vi "Main.vi"(11 "Module Admin":refnum<class "Delacor_lib_QMH_Module Admin.lvclass">) -> ()   [LabVIEW 2019, in "UI.lvlib"]
doc: "This template is based off of the Queued Message Handler design pattern and the Queued Message Handler project template that ships with LabVIEW.\n\nThe main difference is that the queue is private to this module and communication between modules is performed via Broadcast and Request events.\n\nRequest events are wrapped in public API methods and are handled in the Event Handling Loop (EHL) of this VI. Any module can register for Broadcast events sent by this module. The EHL generates messages based on user interface actions.\n\nThe Message Handling Loop (MHL) processes messages generated by the EHL, or by other messages. The messages are string values, so new messages can be added easily to the Message Cases case structure in the MHL. Each message cluster can also provide an optional value for Message Data, which is a variant that can be converted to whatever message-specific data is required.\n_____\nBased on Delacor QMH Project Template 5.0.0.82."
uses:
  UI.lvlib
  <vilib>/Delacor/Delacor QMH/Libraries/Module Admin_class/Delacor_lib_QMH_Module Admin.lvclass
  Module Data--cluster.ctl
  Stop Argument--cluster.ctl
  <vilib>/Delacor/Delacor QMH/Libraries/Message Queue_class/Delacor_lib_QMH_Message Queue.lvclass/Delacor_lib_QMH_Message Queue.ctl
  <vilib>/Delacor/Delacor QMH/Libraries/Module Admin_class/Delacor_lib_QMH_Module Admin.lvclass/Delacor_lib_QMH_Module Admin.ctl
  <vilib>/Delacor/Delacor QMH/Libraries/Message Queue_class/Delacor_lib_QMH_Enqueue Message (Single).vi
  <vilib>/Delacor/Delacor QMH/Libraries/Module Admin_class/Delacor_lib_QMH_Get External Launch.vi
  <vilib>/Utility/error.llb/Error Cluster From Error Code.vi
  <vilib>/ErrorRing/Error Ring.xnode
  <vilib>/Delacor/Delacor QMH/Libraries/Message Queue_class/Delacor_lib_QMH_Message Queue.lvclass
  Adquisition/Adquisition.lvlib
  Analisis/Analisis.lvlib
  Mensajes/Mensajes .lvlib
  config/config.lvlib
panel:
  out "error out":errorcluster
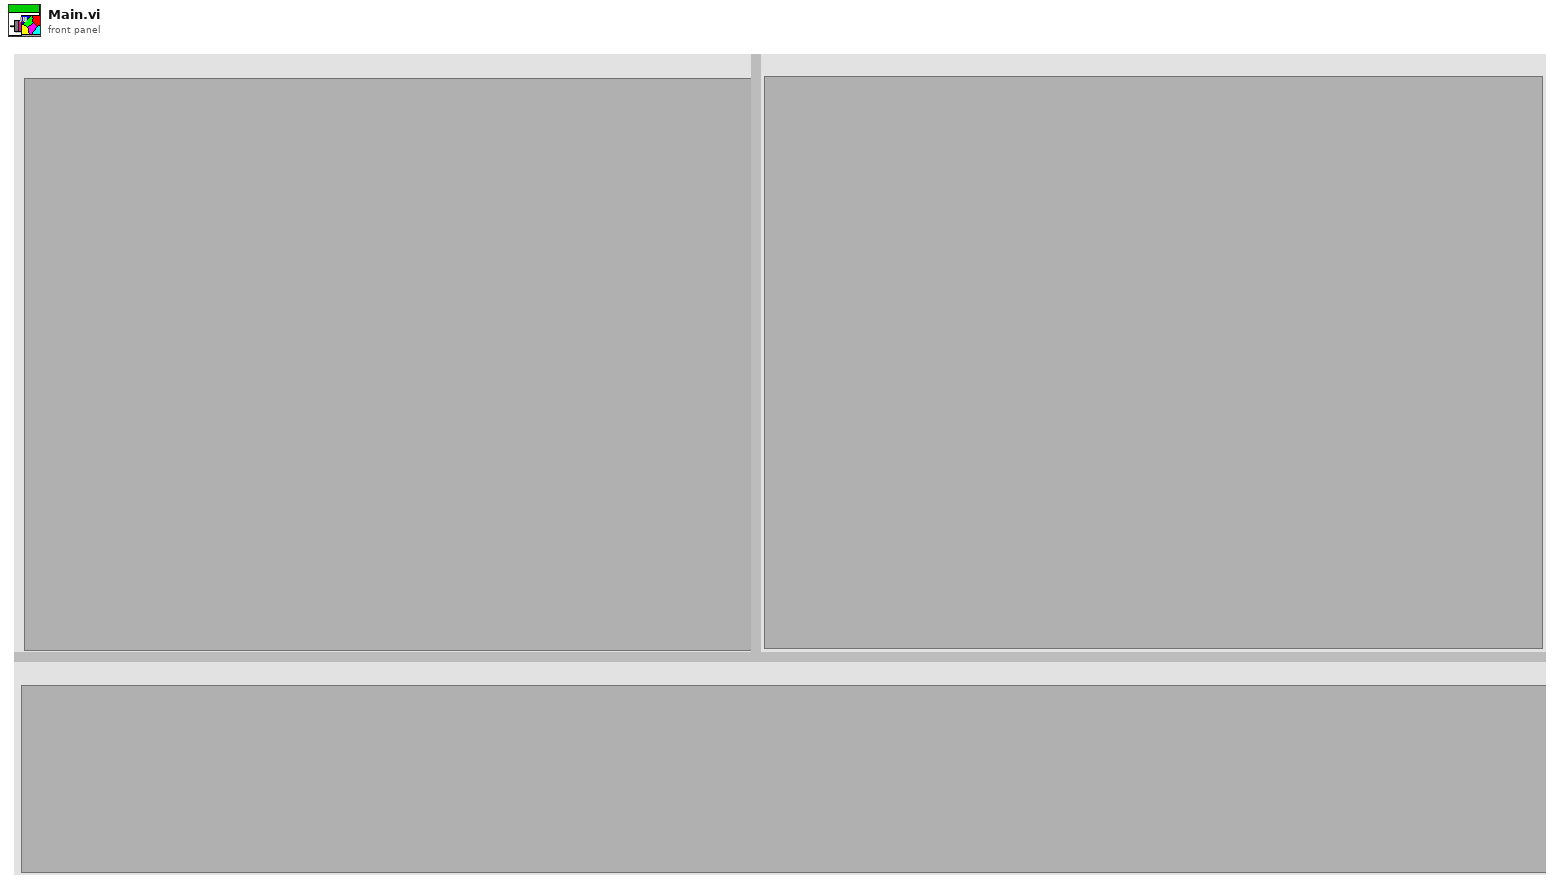
[diagram p1: front panel]
types:
  T1 = typedef "Mensajes .lvlib/Broadcast Events--cluster.ctl" = cluster{"Module Did Init":refnum<user-event>, "Status Updated":refnum<user-event>, "Error Reported":refnum<user-event>, "Module Did Stop":refnum<user-event>, "Update Module Execution Status":refnum<user-event>}
  T2 = typedef "config.lvlib/Broadcast Events--cluster.ctl" = cluster{"Module Did Init":refnum<user-event>, "Status Updated":refnum<user-event>, "Error Reported":refnum<user-event>, "Module Did Stop":refnum<user-event>, "Update Module Execution Status":refnum<user-event>}
  T3 = typedef "Adquisition.lvlib/Broadcast Events--cluster.ctl" = cluster{"Module Did Init":refnum<user-event>, "Status Updated":refnum<user-event>, "Error Reported":refnum<user-event>, "Module Did Stop":refnum<user-event>, "Update Module Execution Status":refnum<user-event>}
  T4 = typedef "Analisis.lvlib/Broadcast Events--cluster.ctl" = cluster{"Module Did Init":refnum<user-event>, "Status Updated":refnum<user-event>, "Error Reported":refnum<user-event>, "Module Did Stop":refnum<user-event>, "Update Module Execution Status":refnum<user-event>}
  T5 = typedef "UI.lvlib/Request Events--cluster.ctl" = cluster{"Stop Module":refnum<user-event>, "Show Panel":refnum<user-event>, "Hide Panel":refnum<user-event>, "Get Module Execution Status":refnum<user-event>, "Show Diagram":refnum<user-event>}
  T6 = typedef "UI.lvlib/Module Data--cluster.ctl" = cluster{"Status":string}
  T7 = enum32{"invalid lock state", "Not Locked", "Locked (No Password)", "Password-protected"}
  T8 = typedef "UI.lvlib/Stop Argument--cluster.ctl" = cluster{"Origin":string, "Exit via Stop Module Req?":bool, "Wait for Module to stop?":bool}
  T9 = enum32{"Invalid", "Standard", "Closed", "Hidden", "Minimized", "Maximized"}
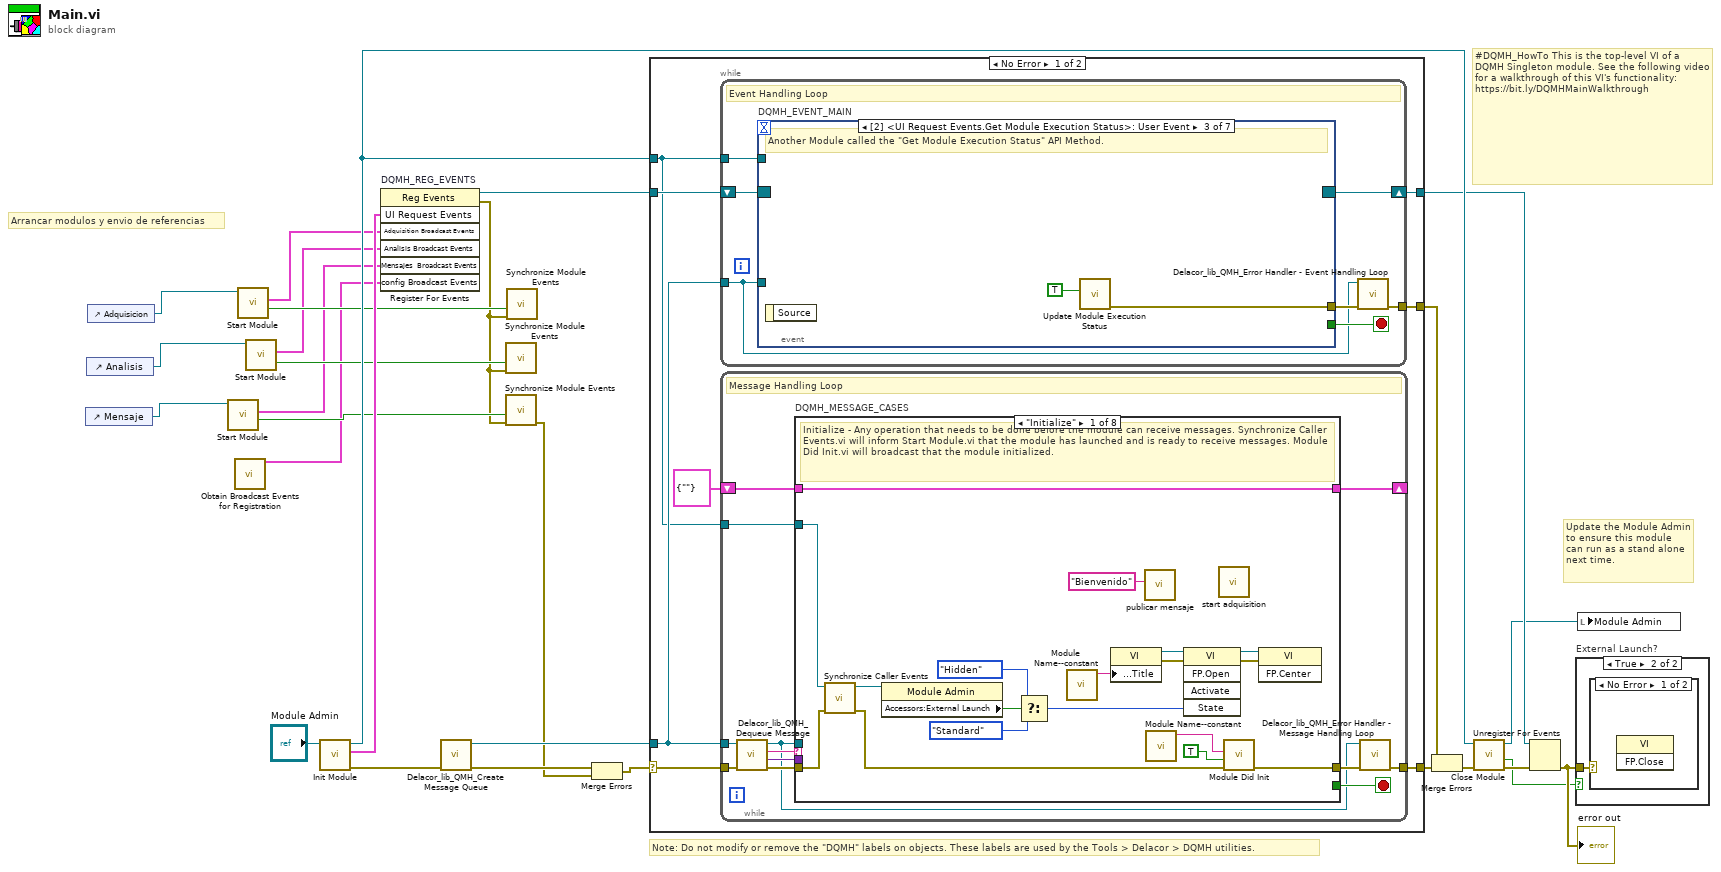
[diagram p0: block diagram]
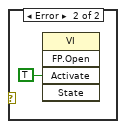
[diagram p3: hidden frame]
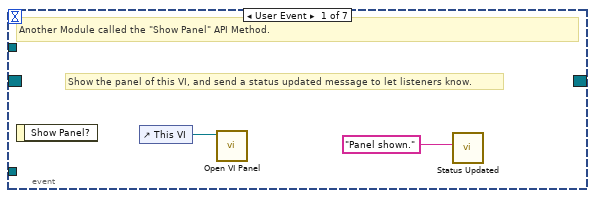
[diagram p4: hidden frame]
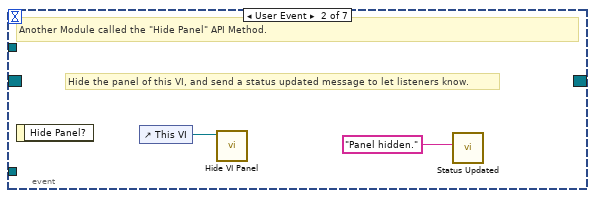
[diagram p5: hidden frame]
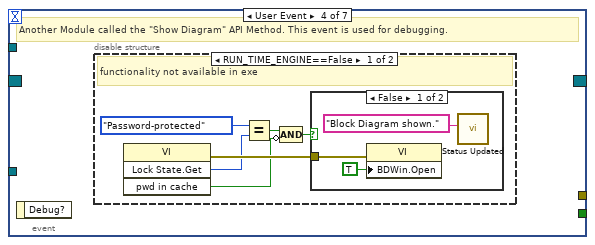
[diagram p6: hidden frame]
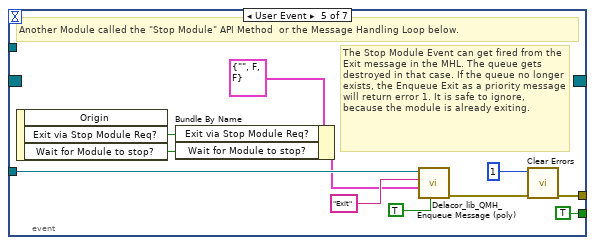
[diagram p9: hidden frame]
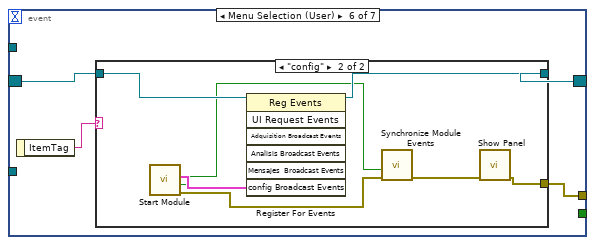
[diagram p10: hidden frame]
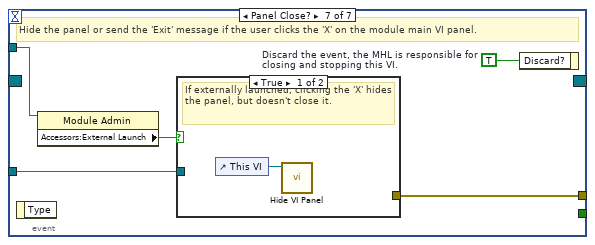
[diagram p12: hidden frame]
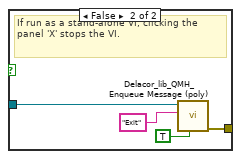
[diagram p13: hidden frame]
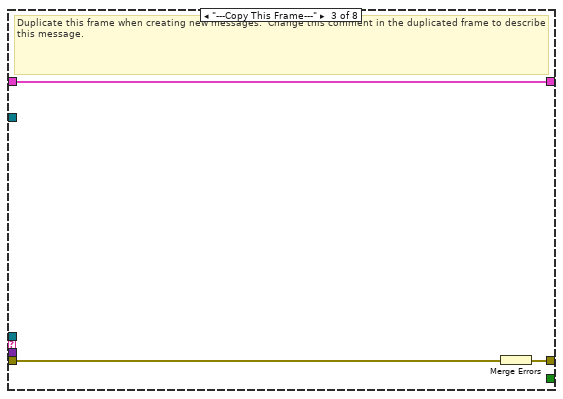
[diagram p15: hidden frame]
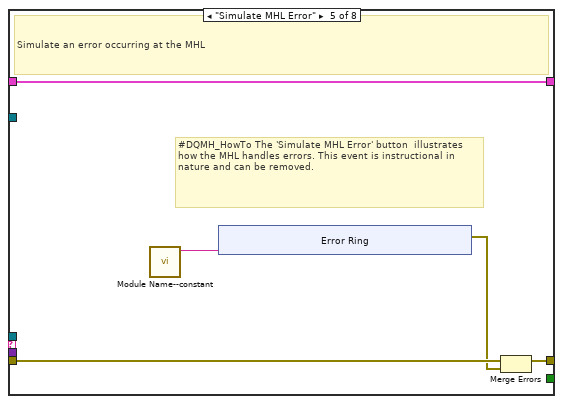
[diagram p17: hidden frame]
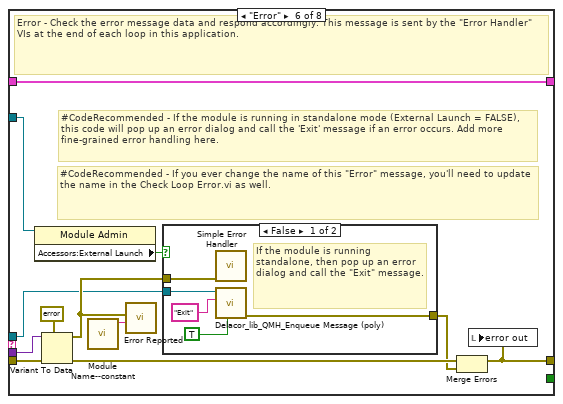
[diagram p18: hidden frame]
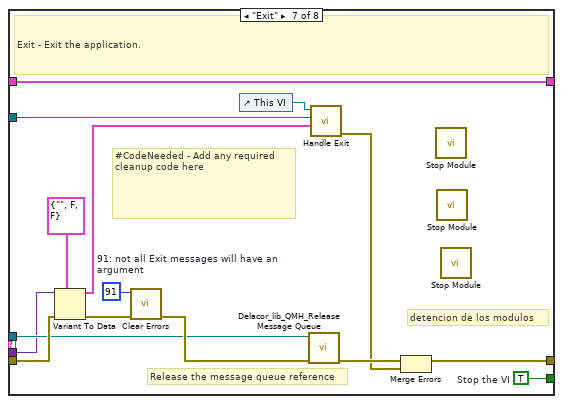
[diagram p20: hidden frame]
diagram:
  # "Arrancar modulos y envio de referencias"
  # "#DQMH_HowTo This is the top-level VI of a DQMH Singleton module. See the following video for a walkthrough of this VI's functionality: https://bit.ly/DQMHMainWalkthrough"
  # "Note: Do not modify or remove the \"DQMH\" labels on objects. These labels are used by the Tools > Delacor > DQMH utilities."
  # "Update the Module Admin to ensure this module can run as a stand alone next time."
  n1 = control-ref of="Mensaje"() -> (w11:refnum<vi>)
  n2 = control-ref of="Analisis"() -> (w12:refnum<vi>)
  n3 = control-ref of="Adquisicion"() -> (w13:refnum<vi>)
  n4 = call "Start Module.vi"("Mensaje"=w11) -> ("Wait for Event Sync?"=w8:bool, "Mensajes  Broadcast Events"=w5:T1)  [unwired: 7 in, 2 out]
  n5 = call "Obtain Broadcast Events for Registration.vi"() -> ("config Broadcast Events"=w1:T2)  [unwired: 9 in, 2 out]
  n6 = call "Start Module.vi"("Adquisicion"=w13) -> ("Wait for Event Sync?"=w10:bool, "Adquisition Broadcast Events"=w7:T3)  [unwired: 7 in, 2 out]
  n7 = call "Start Module.vi"("Analisis"=w12) -> ("Wait for Event Sync?"=w9:bool, "Analisis Broadcast Events"=w6:T4)  [unwired: 7 in, 2 out]
  n8 = call "Init Module.vi"("Singleton Module Admin in"="Module Admin") -> ("error out"=w27:errorcluster, "UI Request Events"=w18:T5, "Singleton Module Admin out"=w21:refnum<class "Delacor_lib_QMH_Module Admin.lvclass">)  [unwired: 8 in]
  n9 = register-events "DQMH_REG_EVENTS"(w18, w7, w6, w5, w1) -> (reference out=w19:refnum<event-registration>, error out=w4:errorcluster)  [unwired: 2 in]
  n10 = call <vilib>:"Delacor_lib_QMH_Create Message Queue.vi"("error in (no error)"=w27) -> ("error out"=w22:errorcluster, "Message Queue"=w17:refnum<class "Delacor_lib_QMH_Message Queue.lvclass">)  [unwired: 9 in]
  n11 = call "Synchronize Module Events.vi"("error in (no error)"=w4, "Wait for Event Sync?"=w9) -> ()  [unwired: 9 in, 1 out]
  n12 = call "Synchronize Module Events.vi"("error in (no error)"=w4, "Wait for Event Sync?"=w8) -> ("error out"=w3:errorcluster)  [unwired: 9 in]
  n13 = call "Synchronize Module Events.vi"("error in (no error)"=w4, "Wait for Event Sync?"=w10) -> ()  [unwired: 9 in, 1 out]
  n14 = Merge Errors(w22, w3) -> (w2:errorcluster)
  n15 = case shown="No Error" w2 {
    selector: w2 -> [w34 w189]
    tunnel: [w36 w188] -> w28
    tunnel: [w33 w194] -> w20
    tunnel: w19 -> [w31 w194]
    tunnel: w17 -> [w30 w187]
    tunnel: [w35 _] -> w25
    tunnel: w21 -> [w29 w190]
    frame No Error {
      n16 = while {
        tunnel: w30 -> [w37]
        shift-right: [w40] -> w33
        shift-left: w31 -> [w41]
        tunnel: [w42] -> w35
        tunnel: w29 -> [w38]
        stop <- w39 stop-if-true
        # "Event Handling Loop"
        n17 = event "DQMH_EVENT_MAIN" shown="[2] <UI Request Events.Get Module Execution Status>: User Event" {
          selector: w41 -> [_ _ _ _ _ w72 _]
          dyn-events: [_ _ _ _ _ w71 _] -> w40
          timeout: _ -> [_ _ _ _ _ _ _]
          tunnel: [_ _ _ _ TRUE ("Discard?") _ _] -> w39
          tunnel: w37 -> [_ _ _ _ w65 _ w84]
          tunnel: [_ _ w49 _ w68 w70 w86] -> w43
          tunnel: w38 -> [_ _ _ _ _ _ w83]
          event User Event {
            # "Show the panel of this VI, and send a status updated message to let listeners know."
            # "Another Module called the \"Show Panel\" API Method."
            n18 = event-data() -> ()  [unwired: 1 in, 1 out]
            n19 = control-ref of="This VI"() -> (w45:refnum<vi>)
            n20 = call "Open VI Panel.vi"("VI"=w45) -> ()  [unwired: 10 in, 1 out]
            n21 = call "Status Updated.vi"("Status"="Panel shown." ("format string")) -> ()  [unwired: 10 in, 1 out]
          }
          event User Event {
            # "Hide the panel of this VI, and send a status updated message to let listeners know."
            # "Another Module called the \"Hide Panel\" API Method."
            n22 = event-data() -> ()  [unwired: 1 in, 1 out]
            n23 = control-ref of="This VI"() -> (w47:refnum<vi>)
            n24 = call "Hide VI Panel.vi"("VI"=w47) -> ()  [unwired: 10 in, 1 out]
            n25 = call "Status Updated.vi"("Status"="Panel hidden." ("format string")) -> ()  [unwired: 10 in, 1 out]
          }
          event User Event {
            # "Another Module called the \"Get Module Execution Status\" API Method."
            n26 = event-data() -> ()  [unwired: 1 in, 1 out]
            n27 = call "Update Module Execution Status.vi"("Running?"=TRUE) -> ("error out"=w49:errorcluster)  [unwired: 10 in]
          }
          event User Event {
            # "Another Module called the \"Show Diagram\" API Method. This event is used for debugging."
            n28 = event-data() -> ()  [unwired: 1 in, 1 out]
            n29 = disable-structure shown="RUN_TIME_ENGINE==False" {
              frame condition #0 (active) {
                # "functionality not available in exe"
                n30 = invoke class="VI" method="Lock State.Get"() -> (error out=w55:errorcluster, "Get Lock State"=w54:T7, "pwd in cache"=w51:bool)  [unwired: 4 in, 1 out]
                n31 = Equal?(x=T7."Password-protected", y=w54) -> (x = y?=w52:bool)
                n32 = Compound Arithmetic op=AND(w52, invert w51) -> (w50:bool)
                n33 = case shown="False" w50 {
                  tunnel: w55 -> [w58 _]
                  frame False {
                    n34 = property class="VI"(error in=w58, "BDWin.Open"=TRUE ("Block Diagram Window:Open")) -> ()  [unwired: 1 in, 2 out]
                    n35 = call "Status Updated.vi"("Status"="Block Diagram shown." ("format string")) -> ()  [unwired: 10 in, 1 out]
                  }
                  frame True {
                    # "Password-protected VI, and the password is not in the cache. Do not show the diagram."
                  }
                }
              }
              frame condition #1 {
              }
            }
          }
          event User Event {
            # "The Stop Module Event can get fired from the Exit message in the MHL. The queue gets destroyed in that case. If the queue no longer exists, the Enqueue Exit as a priority message will return error 1. It is safe to ignore, because the module is already exiting."
            # "Another Module called the \"Stop Module\" API Method  or the Message Handling Loop below."
            n36 = event-data() -> ("Exit via Stop Module Req?"=w61:bool, "Wait for Module to stop?"=w60:bool)  [unwired: 1 in, 1 out]
            n37 = Bundle By Name(cluster=T8 {"Origin"="", "Exit via Stop Module Req?"=FALSE, "Wait for Module to stop?"=FALSE} ("Stop Argument"), "Exit via Stop Module Req?"=w61, "Wait for Module to stop?"=w60) -> (w59:T8)
            n38 = call-poly <vilib>:"Delacor_lib_QMH_Enqueue Message (poly).vi"("Priority Message? (F)"=TRUE, "Message Data"=w59, "Message"="Exit", "Message Queue in"=w65) -> ("error out"=w69:errorcluster)  [unwired: 6 in, 1 out]
            n39 = call <vilib>:"Clear Errors.vi"("error in (no error)"=w69, "specific error code to clear (0: all)"=1) -> ("error out"=w68:errorcluster)  [unwired: 4 in, 1 out]
          }
          event Menu Selection (User) {
            n40 = event-data() -> ("ItemTag"=w73:string)  [unwired: 1 in]
            n41 = case shown="\"config\"" w73 {
              tunnel: w72 -> [w74 w81]
              tunnel: [w74 w80] -> w71
              tunnel: [_ w75] -> w70
              frame "False", Default {
              }
              frame "config" {
                n42 = call "Start Module.vi"() -> ("error out"=w77:errorcluster, "Wait for Event Sync?"=w78:bool, "config Broadcast Events"=w79:T2)  [unwired: 8 in, 1 out]
                n43 = register-events(reference=w81, w79) -> (reference out=w80:refnum<event-registration>)  [unwired: 5 in, 1 out]
                n44 = call "Synchronize Module Events.vi"("error in (no error)"=w77, "Wait for Event Sync?"=w78) -> ("error out"=w76:errorcluster)  [unwired: 9 in]
                n45 = call "Show Panel.vi"("error in (no error)"=w76) -> ("error out"=w75:errorcluster)  [unwired: 10 in]
              }
            }
          }
          event Panel Close? {
            w85 = TRUE  # Discard the event, the MHL is responsible for closing and stopping this VI.
            # "Hide the panel or send the 'Exit' message if the user clicks the 'X' on the module main VI panel."
            n46 = event-data() -> ()  [unwired: 1 in, 1 out]
            n47 = property class="Module Admin"(reference=w83) -> ("Accessors:External Launch"=w82:bool)  [unwired: 1 in, 2 out]
            n48 = case shown="True" w82 {
              tunnel: w84 -> [_ w90]
              tunnel: [_ w91] -> w86
              frame True {
                # "If externally launched, clicking the 'X' hides the panel, but doesn't close it."
                n49 = control-ref of="This VI"() -> (w87:refnum<vi>)
                n50 = call "Hide VI Panel.vi"("VI"=w87) -> ()  [unwired: 10 in, 1 out]
              }
              frame False {
                # "If run as a stand-alone VI, clicking the panel 'X' stops the VI."
                n51 = call-poly <vilib>:"Delacor_lib_QMH_Enqueue Message (poly).vi"("Priority Message? (F)"=TRUE, "Message"="Exit", "Message Queue in"=w90) -> ("error out"=w91:errorcluster)  [unwired: 7 in, 1 out]
              }
            }
            n52 = event-data("Discard?"=w85) -> ()  [unwired: 1 in, 1 out]
          }
        }
        n53 = call-dynamic "Delacor_lib_QMH_Error Handler - Event Handling Loop.vi"("error in (no error)"=w43, "Message Queue in"=w37) -> ("dup error in"=w42:errorcluster)  [unwired: 8 in, 1 out]
      }
      n54 = while {
        tunnel: w30 -> [w94]
        shift-right: [w98] -> _
        shift-left: T6 {"Status"=""} ("Data Cluster") -> [w99]
        tunnel: w34 -> [w102]
        tunnel: [w100] -> w36
        tunnel: w29 -> [w92]
        stop <- w97 stop-if-true
        # "Message Handling Loop"
        n55 = call-dynamic "Delacor_lib_QMH_Dequeue Message.vi"("error in (no error)"=w102, "Message Queue in"=w94) -> ("error out"=w101:errorcluster, "Message Data"=w95:variant, "Message"=w96:string, "Message Queue out"=w93:refnum<class "Delacor_lib_QMH_Message Queue.lvclass">)  [unwired: 6 in]
        n56 = case "DQMH_MESSAGE_CASES" shown="\"Initialize\"" w96 {
          selector: w96 -> [_ _ _ _ _ _ _ w174]
          tunnel: w93 -> [_ _ _ _ _ w144 w166 _]
          tunnel: w101 -> [w119 w123 w126 w128 w133 w151 w172 w176]
          tunnel: [w117 w123 w125 w128 w132 w147 w169 w177] -> w103
          tunnel: w99 -> [w108 w122 w124 w127 w130 w146 w165 w175]
          tunnel: [w108 w122 w124 w127 w130 w146 w165 w175] -> w98
          tunnel: [_ _ _ _ _ _ w164 _] -> w97
          tunnel: w95 -> [_ _ _ _ _ w145 w163 _]
          tunnel: w92 -> [w109 _ _ _ _ w143 w158 _]
          frame "Initialize" {
            # "Initialize - Any operation that needs to be done before the module can receive messages. Synchronize Caller Events.vi will inform Start Module.vi that the module has launched and is ready to receive messages. Module Did Init.vi will broadcast that the module initialized."
            n57 = call "Synchronize Caller Events.vi"("error in (no error)"=w119, "Singleton Module Admin in"=w109) -> ("error out"=w118:errorcluster, "Singleton Module Admin out"=w105:refnum<class "Delacor_lib_QMH_Module Admin.lvclass">)  [unwired: 8 in]
            n58 = property class="Module Admin"(reference=w105) -> ("Accessors:External Launch"=w113:bool)  [unwired: 1 in, 2 out]
            n59 = Select(t=T9."Hidden" ("State"), s=w113, f=T9."Standard" ("State")) -> (s? t:f=w110:T9)
            n60 = call "Module Name--constant.vi"() -> ("Module Name"=w116:string)  [unwired: 11 in]
            n61 = property class="VI"("Front Panel.Title"=w116) -> (reference out=w115:refnum<vi>, error out=w121:errorcluster)  [unwired: 2 in]
            n62 = call "publicar mensaje.vi"("mensaje"="Bienvenido") -> ()  [unwired: 10 in, 1 out]
            n63 = call "Module Name--constant.vi"() -> ("Module Name"=w106:string)  [unwired: 11 in]
            n64 = invoke class="VI" method="FP.Open"(reference=w115, error in=w121, "State"=w110) -> (reference out=w114:refnum<vi>, error out=w120:errorcluster)  [unwired: 2 in, 3 out]
            n65 = call "start adquisition.vi"() -> ()  [unwired: 11 in, 1 out]
            n66 = call "Module Did Init.vi"("error in (no error)"=w118, "Initialized?"=TRUE, "Origin"=w106) -> ("error out"=w117:errorcluster)  [unwired: 8 in]
            n67 = invoke class="VI" method="FP.Center"(reference=w114, error in=w120) -> ()  [unwired: 1 in, 3 out]
          }
          frame "--- Module Specific ---" {
            # "Separator -- The following cases handle messages specific to this Module."
          }
          frame "---Copy This Frame---" {
            # "Duplicate this frame when creating new messages.  Change this comment in the duplicated frame to describe this message."
            n68 = Merge Errors(w126) -> (w125:errorcluster)
          }
          frame "--- Exit and Error Handling---" {
            # "Separator - The following cases handle errors and exit messages."
          }
          frame "Simulate MHL Error" {
            # "#DQMH_HowTo The 'Simulate MHL Error' button  illustrates how the MHL handles errors. This event is instructional in nature and can be removed."
            # "Simulate an error occurring at the MHL"
            n69 = call "Module Name--constant.vi"() -> ("Module Name"=w129:string)  [unwired: 11 in]
            n70 = xnode "Error Ring"("parameter 0"=w129) -> ("error out"=w131:errorcluster)
            n71 = Merge Errors(w133, w131) -> (w132:errorcluster)
          }
          frame "Error" {
            # "#CodeRecommended - If you ever change the name of this \"Error\" message, you'll need to update the name in the Check Loop Error.vi as well."
            # "#CodeRecommended - If the module is running in standalone mode (External Launch = FALSE), this code will pop up an error dialog and call the 'Exit' message if an error occurs. Add more fine-grained error handling here."
            # "Error - Check the error message data and respond accordingly. This message is sent by the \"Error Handler\" VIs at the end of each loop in this application."
            n72 = property class="Module Admin"(reference=w143) -> ("Accessors:External Launch"=w142:bool)  [unwired: 1 in, 2 out]
            n73 = Variant To Data(error in=w151, type=errorcluster {"status"=FALSE, "code"=0, "source"=""} ("error constant"), Variant=w145) -> (data=w152:errorcluster, error out=w149:errorcluster)
            n74 = call "Module Name--constant.vi"() -> ("Module Name"=w141:string)  [unwired: 11 in]
            n75 = call "Error Reported.vi"("Additional Information"=w141, "Error"=w152) -> ()  [unwired: 9 in, 1 out]
            n76 = case shown="False" w142 {
              tunnel: [w157 _] -> w148
              tunnel: w144 -> [w155 _]
              tunnel: w152 -> [w156 _]
              frame False {
                # "If the module is running standalone, then pop up an error dialog and call the \"Exit\" message."
                n77 = call <vilib>:"Simple Error Handler.vi"("error in (no error)"=w156) -> ()  [unwired: 4 in, 5 out]
                n78 = call-poly <vilib>:"Delacor_lib_QMH_Enqueue Message (poly).vi"("Priority Message? (F)"=TRUE, "Message"="Exit", "Message Queue in"=w155) -> ("error out"=w157:errorcluster)  [unwired: 7 in, 1 out]
              }
              frame True {
                # "If the module was launched externally, calling the Error Reported broadcast VI is the only action performed by the \"Error\" message. The module's caller can then process the error appropriately."
              }
            }
            n79 = Merge Errors(w149, w148) -> (w147:errorcluster)
            n80 = local write "error out"(w147) -> ()
          }
          frame "Exit" {
            w162 = 91  # 91: not all Exit messages will have an argument
            w164 = TRUE  # Stop the VI
            # "detencion de los modulos"
            # "Release the message queue reference"
            # "#CodeNeeded - Add any required cleanup code here"
            # "Exit - Exit the application."
            n81 = Variant To Data(error in=w172, type=T8 {"Origin"="", "Exit via Stop Module Req?"=FALSE, "Wait for Module to stop?"=FALSE} ("Stop Argument"), Variant=w163) -> (data=w160:T8, error out=w168:errorcluster)
            n82 = call <vilib>:"Clear Errors.vi"("error in (no error)"=w168, "specific error code to clear (0: all)"=w162) -> ("error out"=w171:errorcluster)  [unwired: 4 in, 1 out]
            n83 = control-ref of="This VI"() -> (w159:refnum<vi>)
            n84 = call-dynamic "Delacor_lib_QMH_Release Message Queue.vi"("error in (no error)"=w171, "Message Queue"=w166) -> ("error out"=w170:errorcluster)  [unwired: 9 in]
            n85 = call "Handle Exit.vi"("Stop Argument"=w160, "Admin in"=w158, "VI reference"=w159) -> ("error out"=w167:errorcluster)  [unwired: 7 in, 1 out]
            n86 = Merge Errors(w170, w167) -> (w169:errorcluster)
            n87 = call "Stop Module.vi"() -> ()  [unwired: 11 in, 1 out]
            n88 = call "Stop Module.vi"() -> ()  [unwired: 11 in, 1 out]
            n89 = call "Stop Module.vi"() -> ()  [unwired: 11 in, 1 out]
          }
          frame Default {
            # "'Default' case only runs if there is a message that isn't defined in any of the other cases.  Output a programming error."
            n90 = call "Module Name--constant.vi"() -> ("Module Name"=w173:string)  [unwired: 11 in]
            n91 = xnode "Error Ring"("parameter 0"=w174, "parameter 1"=w173) -> ("error out"=w178:errorcluster)
            n92 = Merge Errors(w176, w178) -> (w177:errorcluster)
          }
        }
        n93 = call-dynamic "Delacor_lib_QMH_Error Handler - Message Handling Loop.vi"("error in (no error)"=w103, "Message Queue in"=w93) -> ("dup error in"=w100:errorcluster)  [unwired: 8 in, 1 out]
      }
    }
    frame Error {
      # "Synchronize Caller Events.vi will inform Start Module.vi that the module has launched and will let the code calling Start Module.vi register for broadcasts and would permit the caller receive the broadcast that an error occurred at launch time."
      n94 = call-dynamic "Delacor_lib_QMH_Release Message Queue.vi"("error in (no error)"=w189, "Message Queue"=w187) -> ("error out"=w188:errorcluster)  [unwired: 9 in]
      n95 = call "Synchronize Caller Events.vi"("Singleton Module Admin in"=w190) -> ("error out"=w195:errorcluster)  [unwired: 9 in, 1 out]
      n96 = call "Module Name--constant.vi"() -> ("Module Name"=w193:string)  [unwired: 11 in]
      n97 = Format Into String(format string="An error occurred during initialization. %s is no longer running.", w193) -> (resulting string=w191:string)  [unwired: 2 in, 1 out]
      n98 = Merge Errors(w188, w195) -> (w196:errorcluster)
      n99 = call "Error Reported.vi"("Additional Information"=w191, "Error"=w196) -> ()  [unwired: 9 in, 1 out]
    }
  }
  n100 = Merge Errors(w25, w28) -> (w24:errorcluster)
  n101 = call "Close Module.vi"("error in (no error)"=w24, "Module Admin in"=w21) -> ("error out"=w26:errorcluster, "External Launch"=w14:bool, "Module Admin out"=w15:refnum<class "Delacor_lib_QMH_Module Admin.lvclass">)  [unwired: 7 in]
  n102 = Unregister For Events(event registration refnum=w20, error in=w26) -> (error out=w23:errorcluster)
  "error out" <- w23
  n103 = case "External Launch?" shown="True" w14 {
    tunnel: w23 -> [_ w197]
    frame False {
    }
    frame True {
      n104 = case shown="No Error" w197 {
        frame No Error {
          n105 = invoke class="VI" method="FP.Close"() -> ()  [unwired: 3 in, 3 out]
        }
        frame Error {
          n106 = invoke class="VI" method="FP.Open"("Activate"=TRUE ("Activate?")) -> ()  [unwired: 4 in, 5 out]
        }
      }
    }
  }
  n107 = local write "Module Admin"(w15) -> ()
